vi "_Main_LookOnly_V1.1_3el_2021_12_11.vi"() -> ()   [LabVIEW 2017]
uses:
  <vilib>/Instr/_visa.llb/VISA Configure Serial Port (Instr).vi
panel:
  out "Channel 4, V":dbl format="%#_5g"
  in  "DAC 1 LIMIT, V":dbl min=-50.0 max=50.0 format="%#_5g"
  in  "DAC 2, V":dbl min=-10.0 max=10.0 format="%#_5g"
  in  "DAC 1, V":dbl min=-50.0 max=50.0 format="%#_5g"
  out "DAC1volt, V":dbl
  out "Field LOG":cluster{dbl[], dbl[]}(graph)
  out "Bytes at Port":u32
  out "RecTry":i32
  out "Field, kV/cm":dbl
  out "VoltageRes, V":dbl
  out "PlotPoints":cluster{"Time":dbl[], "Voltage":dbl[]}(graph)={"Time"=[0.0, 0.00037111111108161925, 0.000510833333311085, 0.0006505555555405509, 0.0007766666666915019, 0.0009172222221968695, 0.0010569444444263353, 0.0011958333333152243, 0.0013350000000274223], "Voltage"=[5.89, 5.89, 5.89, 5.89, 5.89, 5.89, 5.89, 5.89, 5.89]}
  out "VoltageBelow, V":dbl
  out "Current, mA":dbl format="%#_4g"
  out "Channel 3, V":dbl format="%#_5g"
  out "Channel 2, V":dbl format="%#_5g"
  out "Channel 1, V":dbl format="%#_5g"
  in  "Stop Button":bool
  in  "Start Button":bool
  in  "film H, nm":dbl=50.0
  in  "COM port":refnum<visa-resource-name>
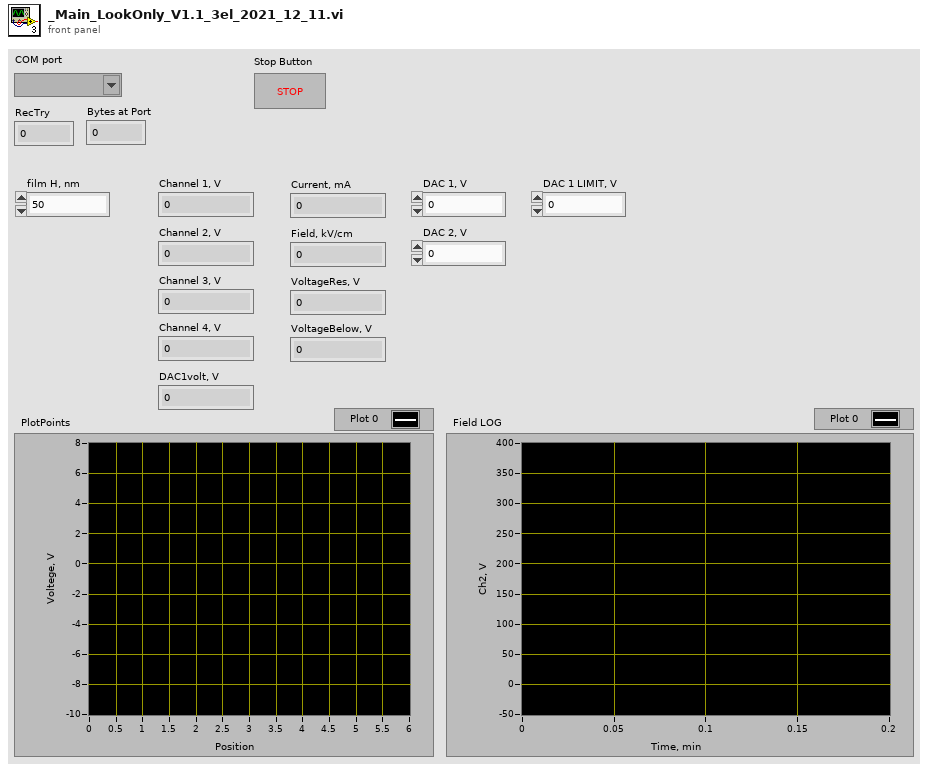
[diagram p1: front panel]
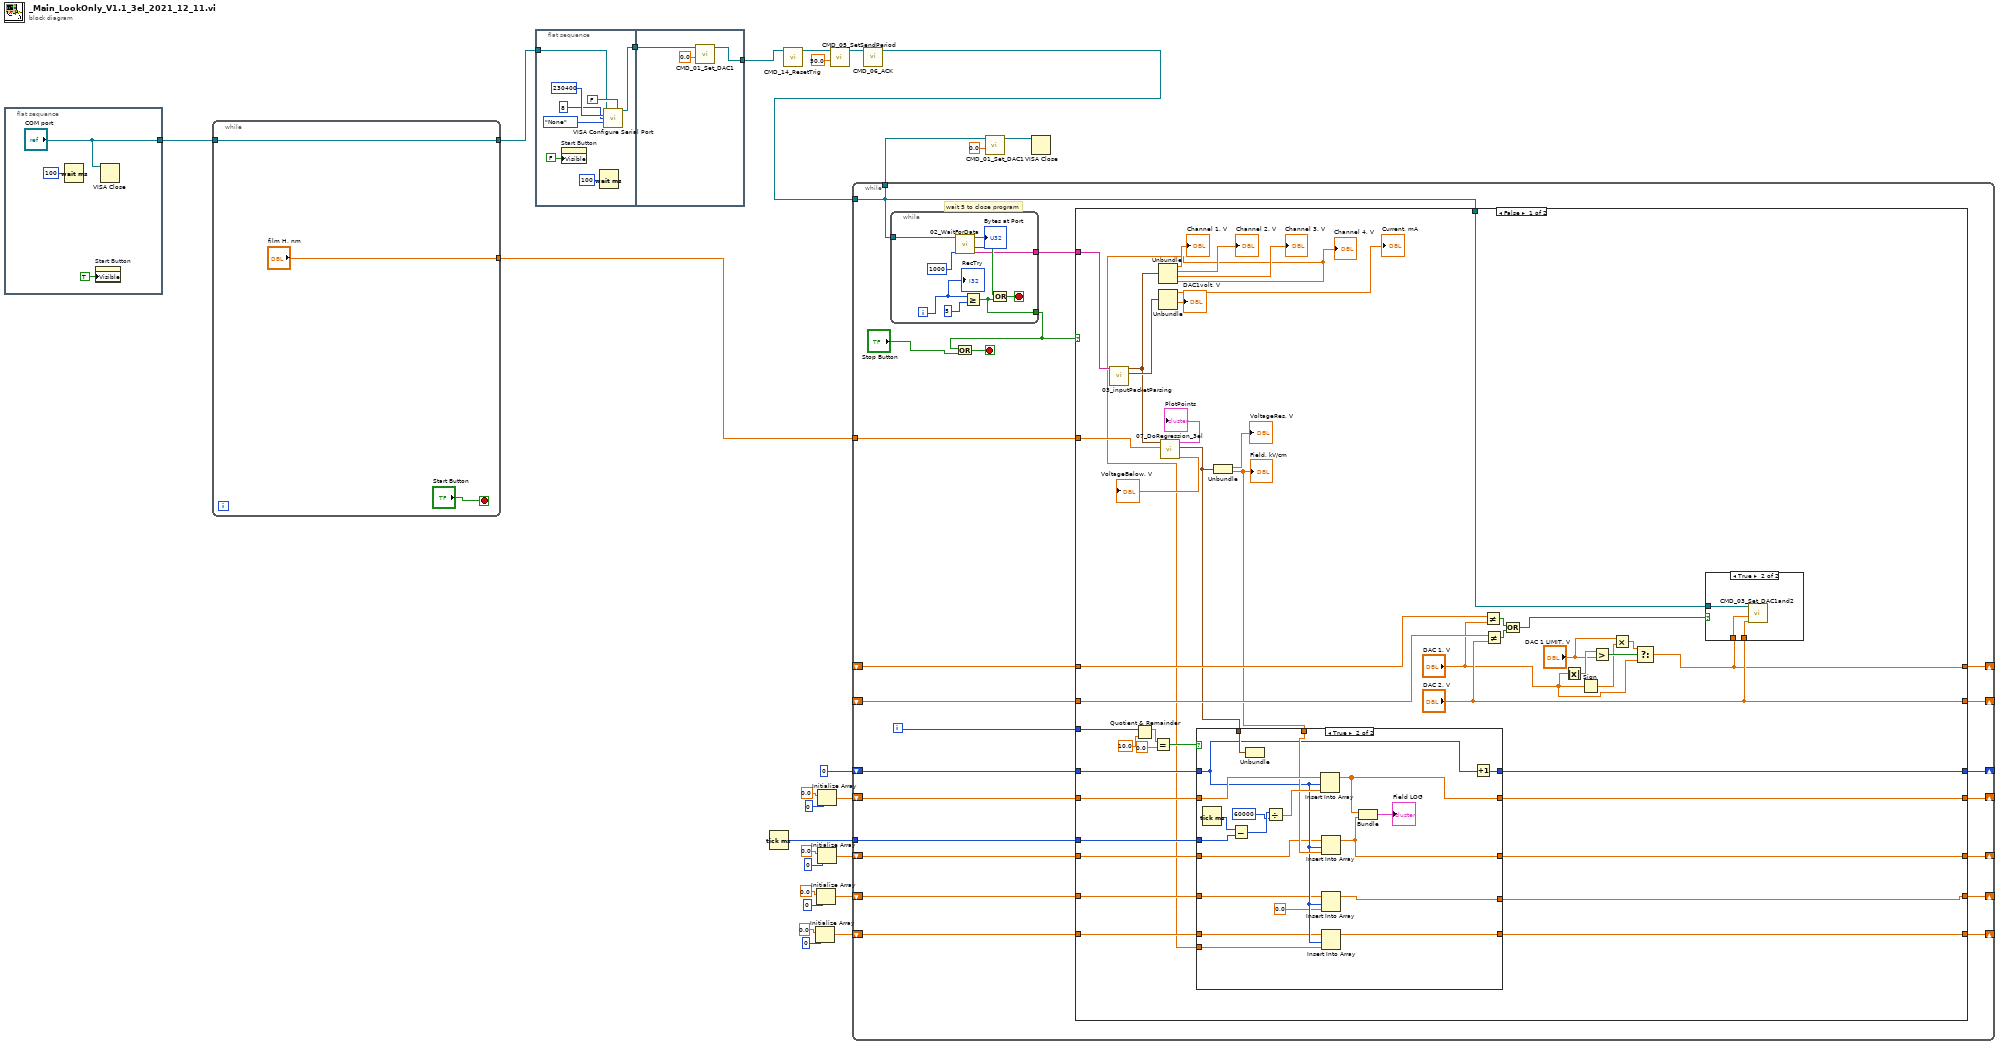
[diagram p0: block diagram]
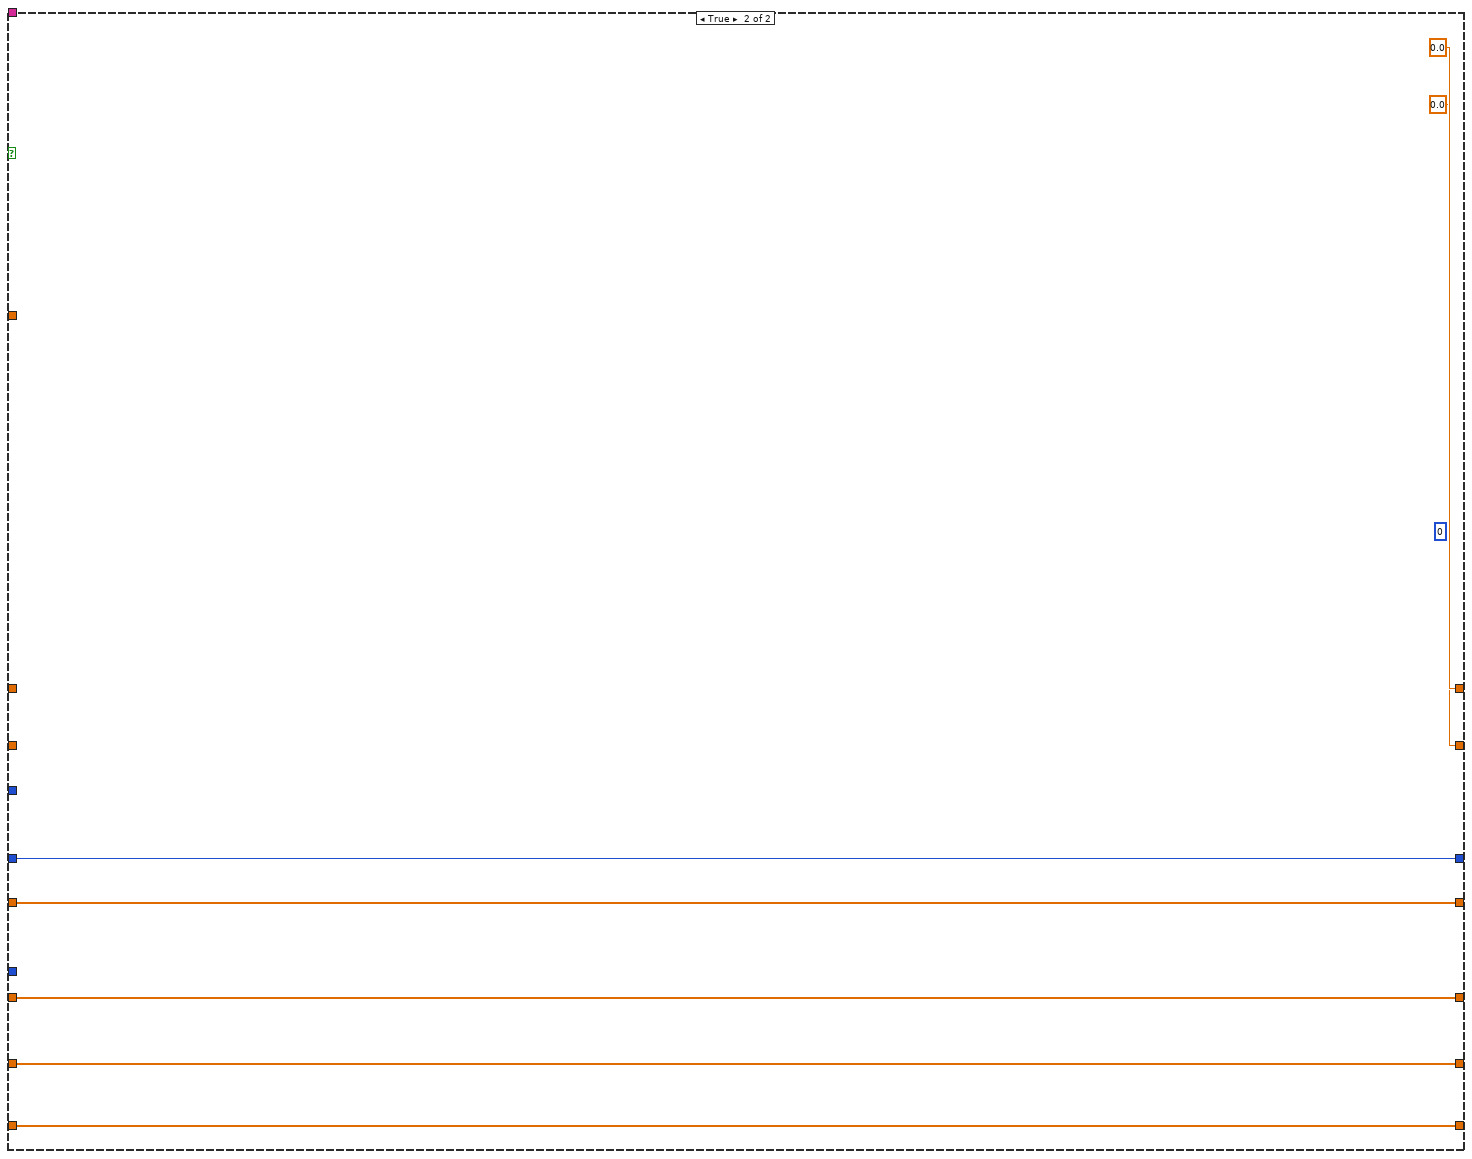
[diagram p4: hidden frame]
diagram:
  n1 = flat-sequence {
    tunnel: ["COM port"] -> w26
    frame #0 {
      n2 = Wait (ms)(milliseconds to wait=u32 100) -> ()  [unwired: 1 out]
      n3 = property on="Start Button" class="Bool"("Visible"=TRUE) -> ()  [unwired: 2 in, 2 out]
      n4 = VISA Close(VISA resource name="COM port") -> ()  [unwired: 1 in, 1 out]
    }
  }
  n5 = while {
    tunnel: w26 -> [w31]
    tunnel: [w31] -> w25
    tunnel: ["film H, nm"] -> w24
    stop <- "Start Button" stop-if-true
  }
  n6 = flat-sequence {
    tunnel: w25 -> [w36]
    tunnel: [w35] -> w15
    tunnel: [w43] -> w22
    tunnel: w15 -> [w42]
    frame #0 {
      n7 = property on="Start Button" class="Bool"("Visible"=FALSE) -> ()  [unwired: 2 in, 2 out]
      n8 = Wait (ms)(milliseconds to wait=u32 100) -> ()  [unwired: 1 out]
      n9 = call-poly "VISA Configure Serial Port"("VISA resource name"=w36, "Enable Termination\nChar (T)"=FALSE ("Enable Termination\nChar (T)"), "baud rate (9600)"=u32 230400, "data bits (8)"=u16 8, "parity (0:none)"=enum16{"None", "Odd", "Even", "Mark", "Space"}."None") -> ("VISA resource name out"=w35:refnum<visa-resource-name>)  [unwired: 9 in, 1 out]
    }
    frame #1 {
      n10 = call "CMD_01_Set_DAC1.vi"("Input, V"=0.0, "VISA resource name"=w42) -> ("VISA resource name out"=w43:refnum<visa-resource-name>)  [unwired: 9 in]
    }
  }
  n11 = Tick Count (ms)() -> (millisecond timer value=w10:u32)
  n12 = call "CMD_14_ResetTrig.vi"("VISA resource name"=w22) -> ("VISA resource name out"=w18:refnum<visa-resource-name>)  [unwired: 10 in]
  n13 = Initialize Array(0.0 ("element"), 0 ("dimension size")) -> (w1:dbl[])
  n14 = Initialize Array(0.0 ("element"), 0 ("dimension size")) -> (w2:dbl[])
  n15 = Initialize Array(0.0 ("element"), 0 ("dimension size")) -> (w7:dbl[])
  n16 = Initialize Array(0.0 ("element"), 0 ("dimension size")) -> (w11:dbl[])
  n17 = call "CMD_05_SetSendPeriod.vi"("Period, ms"=50.0, "VISA resource name"=w18) -> ("VISA resource name out"=w17:refnum<visa-resource-name>)  [unwired: 9 in]
  n18 = call "CMD_06_ACK.vi"("VISA resource name"=w17) -> ("VISA resource name out"=w16:refnum<visa-resource-name>)  [unwired: 10 in]
  n19 = while {
    tunnel: w16 -> [w60]
    tunnel: [w60] -> w23
    tunnel: w24 -> [w62]
    shift-right: [w58] -> _
    shift-left: 0 -> [w59]
    tunnel: w10 -> [w56]
    shift-right: [w54] -> _
    shift-left: w11 -> [w57]
    shift-right: [w53] -> _
    shift-left: w7 -> [w55]
    shift-right: [w51] -> _
    shift-left: _ -> [w48]
    shift-right: [w50] -> _
    shift-left: _ -> [w49]
    shift-right: [w45] -> _
    shift-left: w2 -> [w47]
    shift-right: [w44] -> _
    shift-left: w1 -> [w46]
    i -> [w61]
    stop <- w65 stop-if-true
    # "wait 5 to close program"
    n20 = while {
      tunnel: w60 -> [w146]
      tunnel: [w149] -> w64
      tunnel: [w150] -> w63
      i -> [w148]
      stop <- w152 stop-if-true
      n21 = call "02_WaitForData.vi"("WaitTimeoutMS"=u32 1000, "VISA"=w146) -> ("Buffer"=w150:string, "Bytes at Port"=→"Bytes at Port":u32, "Data Recived"=w151:bool)  [unwired: 7 in]
      n22 = Greater Or Equal?(x=w148, y=5) -> (x >= y?=w149:bool)
      n23 = Or(x=w151, y=w149) -> (x .or. y?=w152:bool)
      "RecTry" <- w148
    }
    n24 = Or(x=w64, y="Stop Button") -> (x .or. y?=w65:bool)
    n25 = case shown="False" w64 {
      tunnel: w63 -> [w110 _]
      tunnel: w62 -> [w76 _]
      tunnel: w61 -> [w103 _]
      tunnel: w60 -> [w86 _]
      tunnel: w59 -> [w101 w145]
      tunnel: [w100 w145] -> w58
      tunnel: w57 -> [w99 w144]
      tunnel: w56 -> [w98 _]
      tunnel: w55 -> [w97 w143]
      tunnel: [w95 w144] -> w54
      tunnel: [w94 w143] -> w53
      tunnel: [w80 0.0 ("DAC 1, V")] -> w51
      tunnel: ["DAC 2, V" 0.0 ("DAC 2, V")] -> w50
      tunnel: w49 -> [w90 _]
      tunnel: w48 -> [w89 _]
      tunnel: w47 -> [w72 w140]
      tunnel: w46 -> [w71 w139]
      tunnel: [w70 w140] -> w45
      tunnel: [w69 w139] -> w44
      frame False {
        n26 = call "03_inputPacketParsing.vi"("string"=w110) -> ("DAC state"=w108:cluster{dbl, dbl, dbl, dbl}, "Voltage"=w75:cluster{dbl, dbl, dbl, dbl})  [unwired: 6 in, 3 out]
        n27 = Quotient & Remainder(x=w103, y=10.0) -> (x-y*floor(x/y)=w106:dbl)  [unwired: 1 out]
        n28 = Equal?(x=w106, y=0.0) -> (x = y?=w102:bool)
        n29 = Unbundle(w75) -> (→"Channel 1, V":dbl, →"Channel 2, V":dbl, →"Channel 3, V":dbl, w66:dbl)
        "Channel 4, V" <- w66
        n30 = Unbundle(w108) -> (→"Current, mA":dbl, →"DAC1volt, V":dbl)  [unwired: 2 out]
        n31 = call "07_DoRegression_3el.vi"("film H, nm"=w76, "Input ChVoltage"=w75) -> ("VoltageBelow, V"=→"VoltageBelow, V":dbl, "Regression"=w74:cluster{"VoltageRes, V":dbl, "Field, kV/cm":dbl}, "PlotPoints"=→"PlotPoints":cluster{"Time":dbl[], "Voltage":dbl[]})  [unwired: 7 in]
        n32 = Unbundle(w74) -> ("VoltageRes, V"=→"VoltageRes, V":dbl, "Field, kV/cm"=w78:dbl)
        "Field, kV/cm" <- w78
        n33 = case shown="True" w102 {
          tunnel: w101 -> [w118 w128]
          tunnel: [w118 w133] -> w100
          tunnel: w74 -> [_ w138]
          tunnel: w99 -> [w116 w131]
          tunnel: w98 -> [_ w136]
          tunnel: w97 -> [w117 w127]
          tunnel: [w117 w123] -> w94
          tunnel: [w116 w130] -> w95
          tunnel: w78 -> [_ w129]
          tunnel: w72 -> [w115 w126]
          tunnel: w71 -> [w114 w125]
          tunnel: [w115 w121] -> w70
          tunnel: [w114 w122] -> w69
          tunnel: w66 -> [_ w124]
          frame False {
          }
          frame True {
            n34 = Tick Count (ms)() -> (millisecond timer value=w137:u32)
            n35 = Subtract(x=w137, y=w136) -> (x-y=w135:u32)
            n36 = Unbundle(w138) -> ()  [unwired: 2 out]
            n37 = Divide(x=w135, y=u32 60000) -> (x/y=w132:dbl)
            n38 = Insert Into Array(array=w131, index=w128, new element=w132) -> (w130:dbl[])
            n39 = Insert Into Array(array=w127, index=w128, new element=w129) -> (w123:dbl[])
            n40 = Insert Into Array(array=w126, index=w128, new element=0.0 ("new element/subarray")) -> (w121:dbl[])
            n41 = Insert Into Array(array=w125, index=w128, new element=w124) -> (w122:dbl[])
            n42 = Bundle(w130, w123) -> (→"Field LOG":cluster{dbl[], dbl[]})  [unwired: 1 in]
            n43 = Increment(x=w128) -> (x+1=w133:i32)
          }
        }
        n44 = Not Equal?(x=w89, y="DAC 1, V") -> (x != y?=w92:bool)
        n45 = Not Equal?(x=w90, y="DAC 2, V") -> (x != y?=w91:bool)
        n46 = Or(x=w92, y=w91) -> (x .or. y?=w88:bool)
        n47 = Absolute Value(x="DAC 1, V") -> (abs(x)=w85:dbl)
        n48 = Sign(1:"DAC 1, V") -> (0:w82:dbl)
        n49 = Greater?(x=w85, y="DAC 1 LIMIT, V") -> (0:w84:bool)
        n50 = Multiply(x="DAC 1 LIMIT, V", y=w82) -> (x*y=w83:dbl)
        n51 = Select(t=w83, s=w84, f="DAC 1, V") -> (s? t:f=w80:dbl)
        n52 = case shown="True" w88 {
          tunnel: "DAC 2, V" -> [_ w113]
          tunnel: w80 -> [_ w112]
          tunnel: w86 -> [_ w111]
          frame False {
          }
          frame True {
            n53 = call "CMD_03_Set_DAC1and2.vi"("Input2, V"=w113, "Input1, V"=w112, "VISA resource name"=w111) -> ()  [unwired: 8 in, 1 out]
          }
        }
      }
      frame True {
        (unwired) u32 0
      }
    }
  }
  n54 = call "CMD_01_Set_DAC1.vi"("Input, V"=0.0, "VISA resource name"=w23) -> ("VISA resource name out"=w20:refnum<visa-resource-name>)  [unwired: 9 in]
  n55 = VISA Close(VISA resource name=w20) -> ()  [unwired: 1 in, 1 out]
